vi "Gwinstek_chan_1_2_sub.vi"(4 "Chan 2":bool, 5 "time":dbl, 6 "DC Offset chan1":dbl, 7 "Enable Output":bool=TRUE, 8 "error in (no error)":errorcluster, 9 "Frequency chan1":dbl=1000.0, 10 "Vpp chan 1":dbl=0.1, 11 "VISA resource name":refnum<visa-resource-name>="COM18") -> (0 "error out":errorcluster, 3 "VISA resource name out":refnum<visa-resource-name>)   [LabVIEW 2018]
uses:
  Downloads/LVdriver_AFG-2225_V1_E/AFG-2225/AFG-2225.lvlib
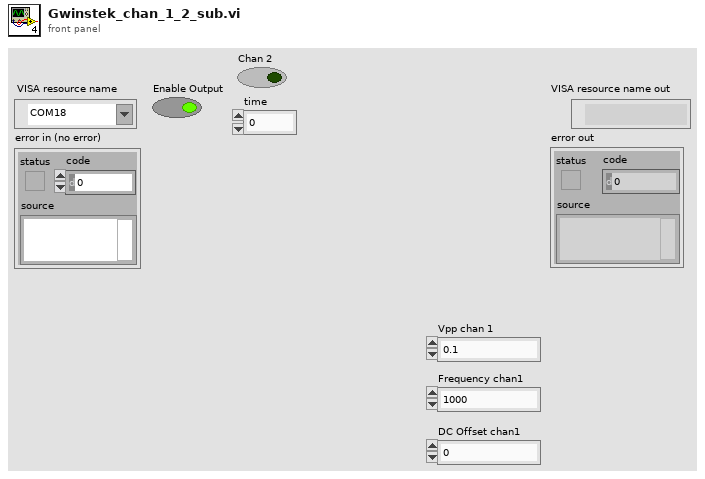
[diagram p1: front panel]
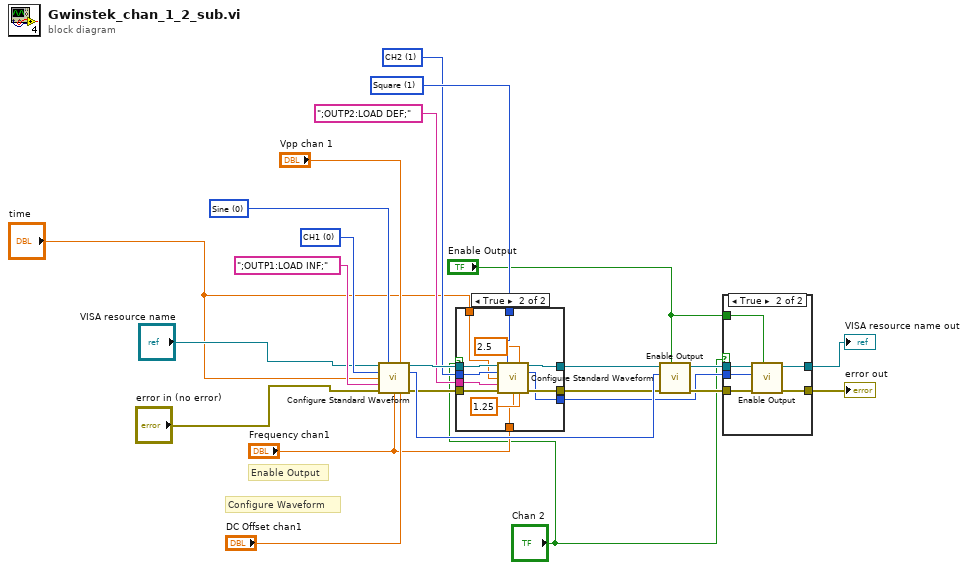
[diagram p0: block diagram]
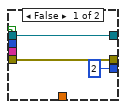
[diagram p3: hidden frame]
diagram:
  w24 = u16 0 items=["Sine", "Square", "Triangle"] ("Waveform chan1")
  w15 = u16 1 items=["Sine", "Square", "Pulse", "Ramp", "Noise"] ("Waveform Function chan2")
  w12 = u16 1 items=["CH1", "CH2"] ("Channel (0: CH1)")
  w21 = u16 0 items=["CH1", "CH2"] ("Channel (0: CH1)")
  # "Enable Output"
  # "Configure Waveform"
  n1 = call "Configure Standard Waveform.vi"("VISA resource name"="VISA resource name", "Waveform Function (0: Sine)"=w24, "Amplitude (3.000 Vpp)"="Vpp chan 1", "Channel (0: CH1)"=w21, "time"="time", "Offset Command"=";OUTP1:LOAD INF;" ("LOAD Command chan 1"), "error in (no error)"="error in (no error)", "Frequency (1000.000 Hz)"="Frequency chan1", "DC Offset (0.00 V)"="DC Offset chan1") -> ("VISA resource name out"=w20:refnum<visa-resource-name>, "Channel out"=w22:u16, "error out"=w17:errorcluster)  [unwired: 4 in]
  n2 = case shown="True" "Chan 2" {
    tunnel: w20 -> [w26 w39]
    tunnel: [w26 w38] -> w19
    tunnel: [w27 w37] -> w18
    tunnel: w17 -> [w27 w36]
    tunnel: w15 -> [_ w35]
    tunnel: w12 -> [_ w33]
    tunnel: ";OUTP2:LOAD DEF;" ("LOAD Command chan 2") -> [_ w31]
    tunnel: "Frequency chan1" -> [_ w30]
    tunnel: [u16 2 ("Channel out") w29] -> w5
    tunnel: "time" -> [_ w28]
    frame False {
    }
    frame True {
      n3 = call "Configure Standard Waveform.vi"("VISA resource name"=w39, "Waveform Function (0: Sine)"=w35, "Amplitude (3.000 Vpp)"=2.5 ("Vpp chan 2"), "Channel (0: CH1)"=w33, "time"=w28, "Offset Command"=w31, "error in (no error)"=w36, "Frequency (1000.000 Hz)"=w30, "DC Offset (0.00 V)"=1.25 ("DC Offset chan 2")) -> ("VISA resource name out"=w38:refnum<visa-resource-name>, "Channel out"=w29:u16, "error out"=w37:errorcluster)  [unwired: 4 in]
    }
  }
  n4 = call "Enable Output.vi"("Enable Output (T: Enable)"="Enable Output", "error in (no error)"=w18, "Channel (0: CH1)"=w22, "VISA resource name"=w19) -> ("error out"=w13:errorcluster, "VISA resource name out"=w14:refnum<visa-resource-name>)  [unwired: 6 out]
  n5 = case shown="True" "Chan 2" {
    tunnel: w14 -> [w41 w47]
    tunnel: w13 -> [w40 w46]
    tunnel: [w41 w45] -> w8
    tunnel: [w40 w44] -> w7
    tunnel: "Enable Output" -> [_ w43]
    tunnel: w5 -> [_ w42]
    frame False {
    }
    frame True {
      n6 = call "Enable Output.vi"("Enable Output (T: Enable)"=w43, "error in (no error)"=w46, "Channel (0: CH1)"=w42, "VISA resource name"=w47) -> ("error out"=w44:errorcluster, "VISA resource name out"=w45:refnum<visa-resource-name>)  [unwired: 6 out]
    }
  }
  "VISA resource name out" <- w8
  "error out" <- w7
